vi "constructor.vi"(8 "error in (no error)":errorcluster, 11 "deviceName":string) -> (0 "error out":errorcluster, 3 "AnalogOutput out":refnum<class "AnalogOutput.lvclass">)   [LabVIEW 2009, in "Hardware.lvlib" / "Channels.lvlib" / "AnalogOutput.lvclass"]
uses:
  AnalogOutput.lvclass
  niDAQmxAO.lvclass
  SoundAO/SoundAO.lvclass
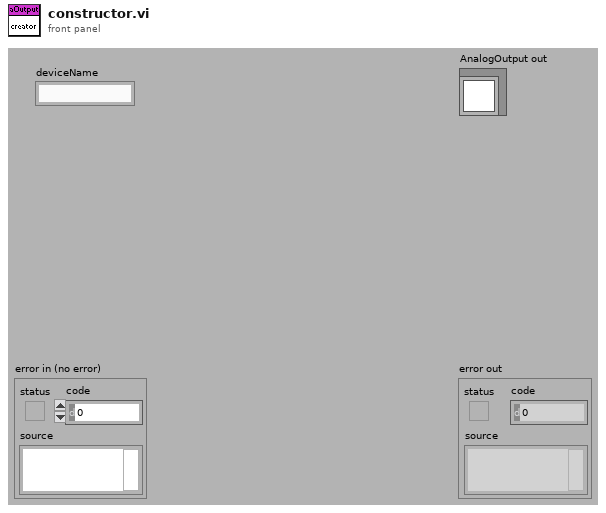
[diagram p1: front panel]
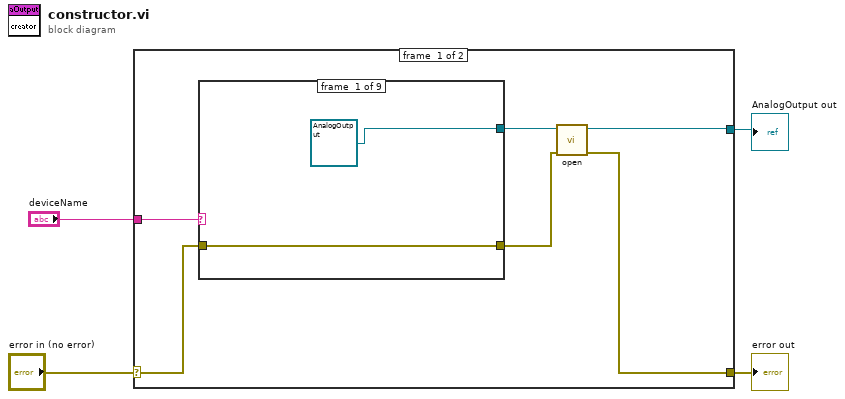
[diagram p0: block diagram]
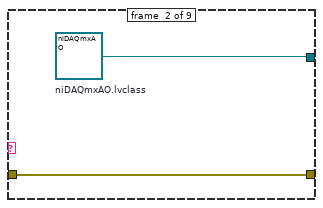
[diagram p2: hidden frame]
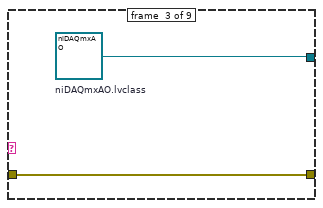
[diagram p3: hidden frame]
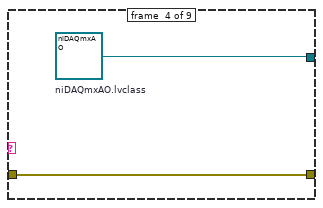
[diagram p4: hidden frame]
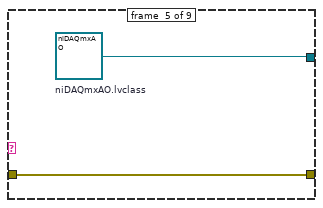
[diagram p5: hidden frame]
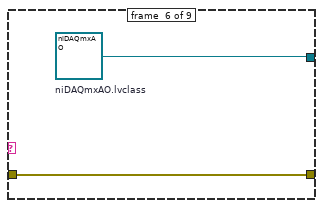
[diagram p6: hidden frame]
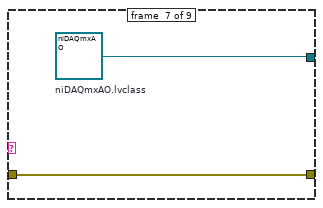
[diagram p7: hidden frame]
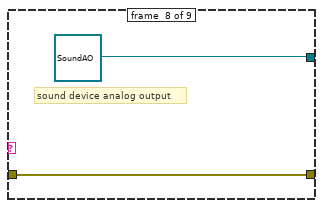
[diagram p8: hidden frame]
diagram:
  n1 = case shown="No Error" "error in (no error)" {
    selector: "error in (no error)" -> [w10 w28]
    tunnel: [w5 w28] -> w3
    tunnel: [w7 _] -> w2
    tunnel: "deviceName" -> [w9 _]
    frame #0 {
      n2 = case shown="\"K2602\"" w9 {
        tunnel: [refnum<class "AnalogOutput.lvclass"> refnum ("Hardware:Channels.lvlib:AnalogOutput.lvclass") w13 w15 w17 w19 w21 w23 refnum<class "SoundAO.lvclass"> refnum ("Hardware:Channels.lvlib:SoundAO.lvclass") _] -> w8
        tunnel: w10 -> [w12 w14 w16 w18 w20 w22 w24 w26 w27]
        tunnel: [w12 w14 w16 w18 w20 w22 w24 w26 w27] -> w6
        frame #0 {
        }
        frame #1 {
          w13 = refnum<class "niDAQmxAO.lvclass"> refnum  # niDAQmxAO.lvclass
        }
        frame #2 {
          w15 = refnum<class "niDAQmxAO.lvclass"> refnum  # niDAQmxAO.lvclass
        }
        frame #3 {
          w17 = refnum<class "niDAQmxAO.lvclass"> refnum  # niDAQmxAO.lvclass
        }
        frame #4 {
          w19 = refnum<class "niDAQmxAO.lvclass"> refnum  # niDAQmxAO.lvclass
        }
        frame #5 {
          w21 = refnum<class "niDAQmxAO.lvclass"> refnum  # niDAQmxAO.lvclass
        }
        frame #6 {
          w23 = refnum<class "niDAQmxAO.lvclass"> refnum  # niDAQmxAO.lvclass
        }
        frame #7 {
          # "sound device analog output"
        }
        frame #8 {
        }
      }
      n3 = call-dynamic "open.vi"("error in (no error)"=w6, "AnalogOutput in"=w8) -> ("error out"=w5:errorcluster, "AnalogOutput out"=w7:refnum<class "AnalogOutput.lvclass">)  [unwired: 8 in]
    }
    frame #1 {
    }
  }
  "error out" <- w3
  "AnalogOutput out" <- w2
